vi "SRS 830 read Channel 1.vi"(2 "Point #":i32, 3 "Instrument Address":refnum<visa-resource-name>) -> (0 "Stop":bool, 1 "SRS 830 Output":dbl[](array[numeric]) format="%.2e")   [LabVIEW 2024]
doc: "This VI reads two channels of the PAR 5210 lockin. It will not work for the 5208. The output is an array of values. The input is the numeric GPIB address.\nScott Hannahs, F. Bitter National Magnet Lab, May 1993"
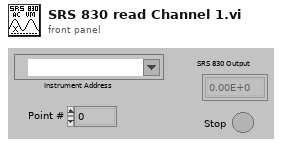
[diagram p1: front panel]
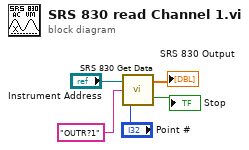
[diagram p0: block diagram]
diagram:
  n1 = call "SRS 830 Get Data.vi"("Point #"="Point #", "Command String"="OUTR?1", "Instrument Address"="Instrument Address") -> ("Stop"=→"Stop":bool, "SRS 830 Output"=→"SRS 830 Output":dbl[])
